vi "get Session Prefix.vi"(7 "Local Listener Session":refnum<class "Local Listener Session.lvclass">) -> (8 "Session Prefix":string)   [LabVIEW 2012, in "REx.lvlib" / "Local Listener Session.lvclass"]
uses:
  Local Listener Session.lvclass
  <userlib>/_Session Fwk/Session - Root.lvclass
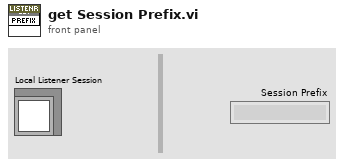
[diagram p1: front panel]
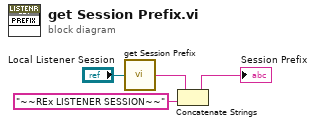
[diagram p0: block diagram]
diagram:
  n1 = call-parent "get Session Prefix.vi"("Session - Root"="Local Listener Session") -> ("Session Prefix"=w3:string)  [unwired: 14 in]
  n2 = Concatenate Strings(w3, "~~REx LISTENER SESSION~~" ("string")) -> (→"Session Prefix":string)
